vi "PhotonPipelineResult_SetTimeStampSecs.vi"(9 "TimeStampSec":dbl, 11 "PhotonPipelineResult_REF":T1) -> (3 "Out PhotonPipelineResult_REF":T1)   [LabVIEW 2019, in "PhotonVisionLib.lvlib"]
doc: "Returns pipeline packet time stamp\n\nInputs:\n - PipelineResult -- Parsed PipelineResult cluster.\n - TimeStampSec -- Time stamp of packet (FPGA elapsed time) seconds\n\nOutputs:\n - Out PipelineResult -- Updated PipelineResult cluster."
uses:
  PhotonVisionLib.lvlib
  TypeDef/TargetCornerType.ctl
  TypeDef/PhotonTrackedTargetType.ctl
  TypeDef/PhotonPipelineResultType.ctl
  <vilib>/Rock Robotics/WPI/ThirdParty/JAS_Junk/TrajLib/TypeDef/TRANSLATION3D.ctl
  <vilib>/Rock Robotics/WPI/ThirdParty/JAS_Junk/TrajLib/Trajectory_Library.lvlib
  <vilib>/Rock Robotics/WPI/ThirdParty/JAS_Junk/TrajLib/TypeDef/QUATERNION.ctl
  <vilib>/Rock Robotics/WPI/ThirdParty/JAS_Junk/TrajLib/TypeDef/ROTATION3D.ctl
  <vilib>/Rock Robotics/WPI/ThirdParty/JAS_Junk/TrajLib/TypeDef/TRANSFORM3D.ctl
  TypeDef/PhotonPNPResultType.ctl
  TypeDef/PhotonMultiTargetPNPResultType.ctl
  Ref/PhotonPipelineResult_REF.ctl
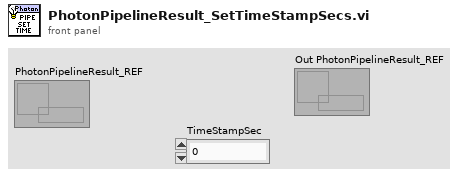
[diagram p1: front panel]
types:
  T1 = typedef "PhotonVisionLib.lvlib/PhotonPipelineResult_REF.ctl" = refnum<data-value>
  T2 = typedef "PhotonVisionLib.lvlib/PhotonPipelineResultType.ctl" = cluster{"TargetCount":i32, "Latency_MilliSec":dbl, "Targets":T3[], "TimeStampSec":dbl, "PhotonMultiTargetPNPResult":T9}
  T3 = typedef "PhotonVisionLib.lvlib/PhotonTrackedTargetType.ctl" = cluster{"Yaw":dbl, "Pitch":dbl, "Area":dbl, "Skew":dbl, "MinAreaRectCorners":T4[], "BestCameraToTarget":T5, "FiiducialId":i32, "AltCameraToTarget":T5, "PoseAmbiguity":dbl, "DetectedCorners":T4[]}
  T4 = typedef "PhotonVisionLib.lvlib/TargetCornerType.ctl" = cluster{"X":dbl, "Y":dbl}
  T5 = typedef "Trajectory_Library.lvlib/TRANSFORM3D.ctl" = cluster{"TRANSLATION3D":T6, "ROTATION3D":T7, "XF":bool}
  T6 = typedef "Trajectory_Library.lvlib/TRANSLATION3D.ctl" = cluster{"X":dbl, "Y":dbl, "Z":dbl}
  T7 = typedef "Trajectory_Library.lvlib/ROTATION3D.ctl" = cluster{"Q_quaternion":T8}
  T8 = typedef "Trajectory_Library.lvlib/QUATERNION.ctl" = cluster{"R":dbl, "V":dbl[]}
  T9 = typedef "PhotonVisionLib.lvlib/PhotonMultiTargetPNPResultType.ctl" = cluster{"PhotonPNPResult":T10, "FiducialIDsUsed":i16[]}
  T10 = typedef "PhotonVisionLib.lvlib/PhotonPNPResultType.ctl" = cluster{"IsPresent":bool, "bestReprojErr":dbl, "altReprojErr":dbl, "ambiguity":dbl, "Best":T5, "Alt":T5}
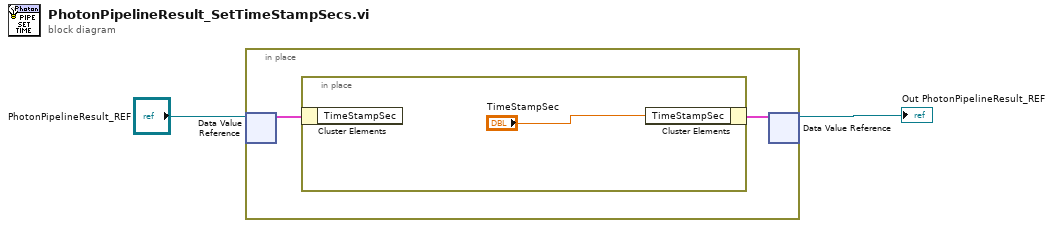
[diagram p0: block diagram]
diagram:
  n1 = in-place {
    n2 = in-place-dvr #1("PhotonPipelineResult_REF") -> (w4:T2)  [unwired: 1 out]
    n3 = in-place {
      n4 = in-place-cluster #2(w4) -> ()  [unwired: 1 out]
      n5 = in-place-cluster #2("TimeStampSec"="TimeStampSec") -> (w3:T2)
    }
    n6 = in-place-dvr #1(w3) -> (→"Out PhotonPipelineResult_REF":T1)  [unwired: 1 out]
  }
